vi "niDTS BT INSTR TX UTIL Average Type IBE.vi"(7 "Outer":T1(ring)) -> (8 "Enum":T2(ring))   [LabVIEW 2015, in "niDTS BT.lvlib" / "niDTS BT INSTR TX.lvclass"]
uses:
  niDTS BT INSTR TX.lvclass
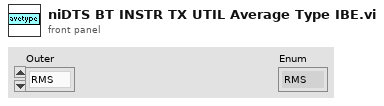
[diagram p1: front panel]
types:
  T1 = enum16{"RMS", "LOG", "SCALAR", "MAX", "MIN", "VECTOR"}
  T2 = enum16{"RMS", "LOG", "SCALar", "MAX", "MIN", "VECTor"}
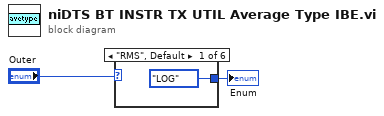
[diagram p0: block diagram]
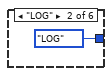
[diagram p2: hidden frame]
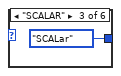
[diagram p3: hidden frame]
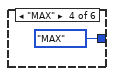
[diagram p4: hidden frame]
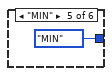
[diagram p5: hidden frame]
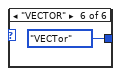
[diagram p6: hidden frame]
diagram:
  n1 = case shown="\"RMS\", Default" "Outer" {
    tunnel: [T2."LOG" T2."LOG" T2."SCALar" T2."MAX" T2."MIN" T2."VECTor"] -> w2
    frame "RMS", Default {
    }
    frame "LOG" {
    }
    frame "SCALAR" {
    }
    frame "MAX" {
    }
    frame "MIN" {
    }
    frame "VECTOR" {
    }
  }
  "Enum" <- w2
